vi "idxArrayToBoolArray.vi"(8 "error in (no error)":errorcluster, 10 "Idx Array":i32[](array[numeric]), 11 "Length of Bool Array":i32) -> (0 "error out":errorcluster, 2 "Bool Array":bool[](array[boolean]))   [LabVIEW 2016]
doc: "Translate the index array to boolean array. (e.g. [0, 2] -> [T, F, T])."
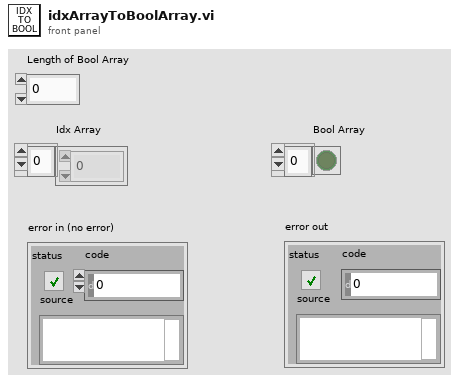
[diagram p1: front panel]
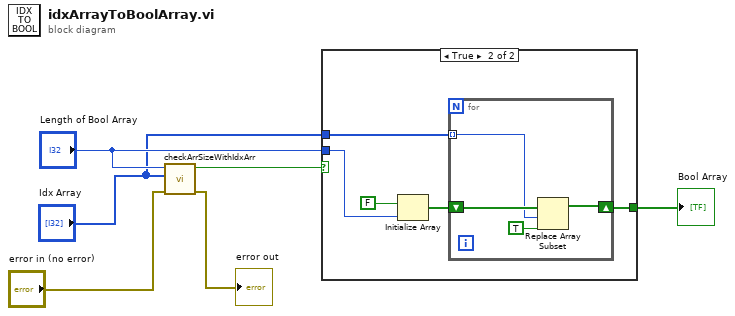
[diagram p0: block diagram]
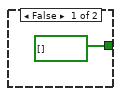
[diagram p2: hidden frame]
diagram:
  n1 = call "checkArrSizeWithIdxArr.vi"("error in (no error)"="error in (no error)", "Idx Array"="Idx Array", "Array Size"="Length of Bool Array") -> ("error out"=→"error out":errorcluster, "In Spec"=w1:bool)  [unwired: 7 in]
  n2 = case shown="True" w1 {
    tunnel: [bool[] [] w10] -> w6
    tunnel: "Length of Bool Array" -> [_ w9]
    tunnel: "Idx Array" -> [_ w8]
    frame False {
    }
    frame True {
      n3 = Initialize Array(FALSE, w9) -> (w11:bool[])
      n4 = for {
        shift-right: [w14] -> w10
        shift-left: w11 -> [w16]
        tunnel: w8 -> [w15] mode=indexing
        n5 = Replace Array Subset(array=w16, new element=TRUE, index=w15) -> (w14:bool[])
      }
    }
  }
  "Bool Array" <- w6
